vi "pop_growth_B.vi"(8 "sat pol in":dbl, 10 "rho - val in":dbl, 11 "rho + val in":dbl) -> (3 "Growth val out":dbl)   [LabVIEW 2018]
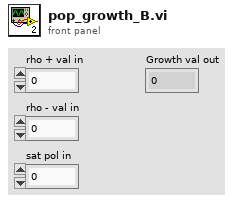
[diagram p1: front panel]
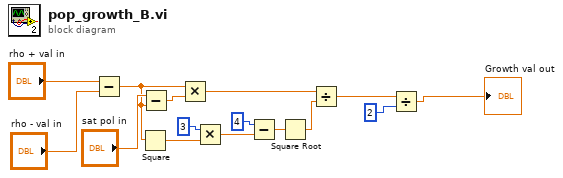
[diagram p0: block diagram]
diagram:
  n1 = Subtract(x="rho + val in", y="rho - val in") -> (x-y=w10:dbl)
  n2 = Square(x=w10) -> (x^2=w8:dbl)
  n3 = Subtract(x="sat pol in", y=w10) -> (x-y=w12:dbl)
  n4 = Multiply(x=w10, y=w12) -> (x*y=w5:dbl)
  n5 = Multiply(x=3, y=w8) -> (x*y=w7:dbl)
  n6 = Subtract(x=4, y=w7) -> (x-y=w6:dbl)
  n7 = Square Root(x=w6) -> (sqrt(x)=w4:dbl)
  n8 = Divide(x=w5, y=w4) -> (x/y=w2:dbl)
  n9 = Divide(x=w2, y=2) -> (x/y=→"Growth val out":dbl)
